vi "数据查询_数据查询.vi"() -> ()   [LabVIEW 2016]
uses:
  <vilib>/Utility/miscctls.llb/LVPointTypeDef.ctl
  <vilib>/Utility/miscctls.llb/LVRowAndColumnUnsignedTypeDef.ctl
  <userlib>/_OpenG.lib/array/array.llb/Sort 2D Array (String)__ogtk.vi
  <userlib>/_OpenG.lib/array/array.llb/Sort 1D Array (I32)__ogtk.vi
  <vilib>/addons/database/_DB Variant To Data/Database Variant To Data.xnode
panel:
  out "布尔文本.文本":string
  in  "数值":dbl=100.0 caption="显示条数"
  in  "单选按钮":T1(radio)
  in  "滚动条":i32(c297)
  in  "数组":string[](array[string])
  in  "导出":bool
  out "数据筛选_分钟小时":string(combo)="实时数据"
  out "数据筛选_工作类型":string(combo)="全部数据"
  out "连接的字符串":string
  out "选中数据表":string
  in  "查询":bool
  in  "结束日期":string="2050/01/01"
  in  "起始日期":string="2010/01/01"
  out "XY图":cluster{"data":timestamp[], "data":dbl[]}[](graph)
  in  "数据表":T2
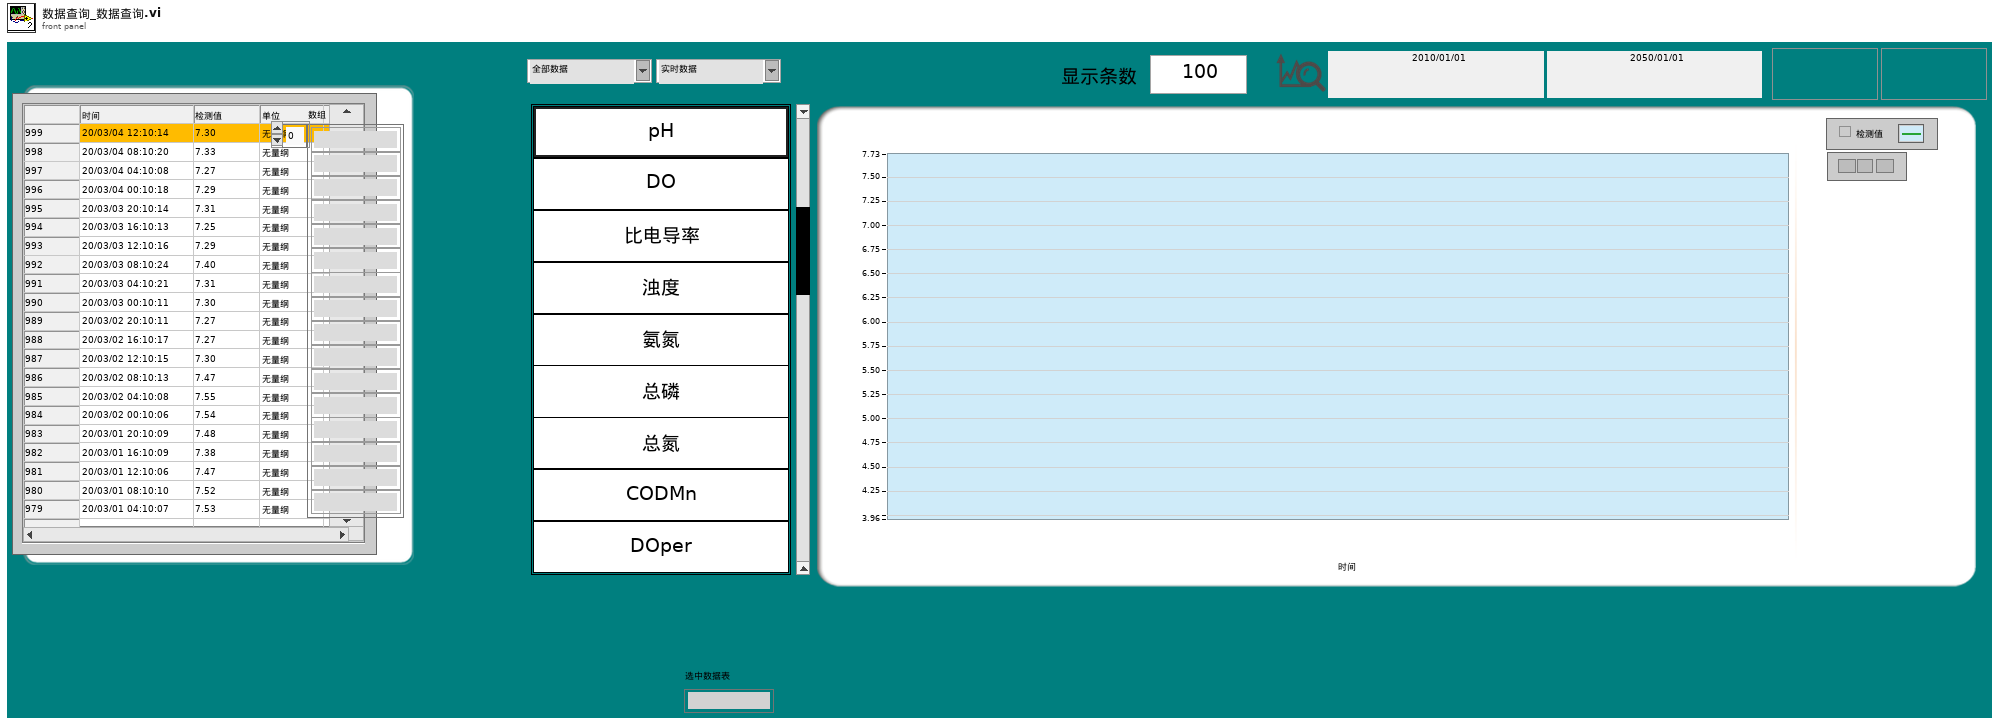
[diagram p1: front panel]
types:
  T1 = enum32{"单选选项1", "单选选项1 2", "单选选项1 3", "单选选项1 4", "单选选项1 5", "单选选项1 6", "单选选项1 7", "单选选项1 8", "单选选项1 9"}
  T2 = typedef "数据查询页列表框.ctl" = i32
  T3 = typedef "LVRowAndColumnUnsignedTypeDef.ctl" = cluster{"Row":u32, "Column":u32}
  T4 = typedef "LVPointTypeDef.ctl" = cluster{"Horizontal":i16, "Vertical":i16}
  T5 = enum8{"Enabled", "Disabled", "Disabled and Grayed Out"}
  T6 = typedef "LVPoint32TypeDef.ctl" = cluster{"Horizontal":i32, "Vertical":i32}
  T7 = typedef "LVPointDoubleTypeDef.ctl" = cluster{"Cursor X":dbl, "Cursor Y":dbl}
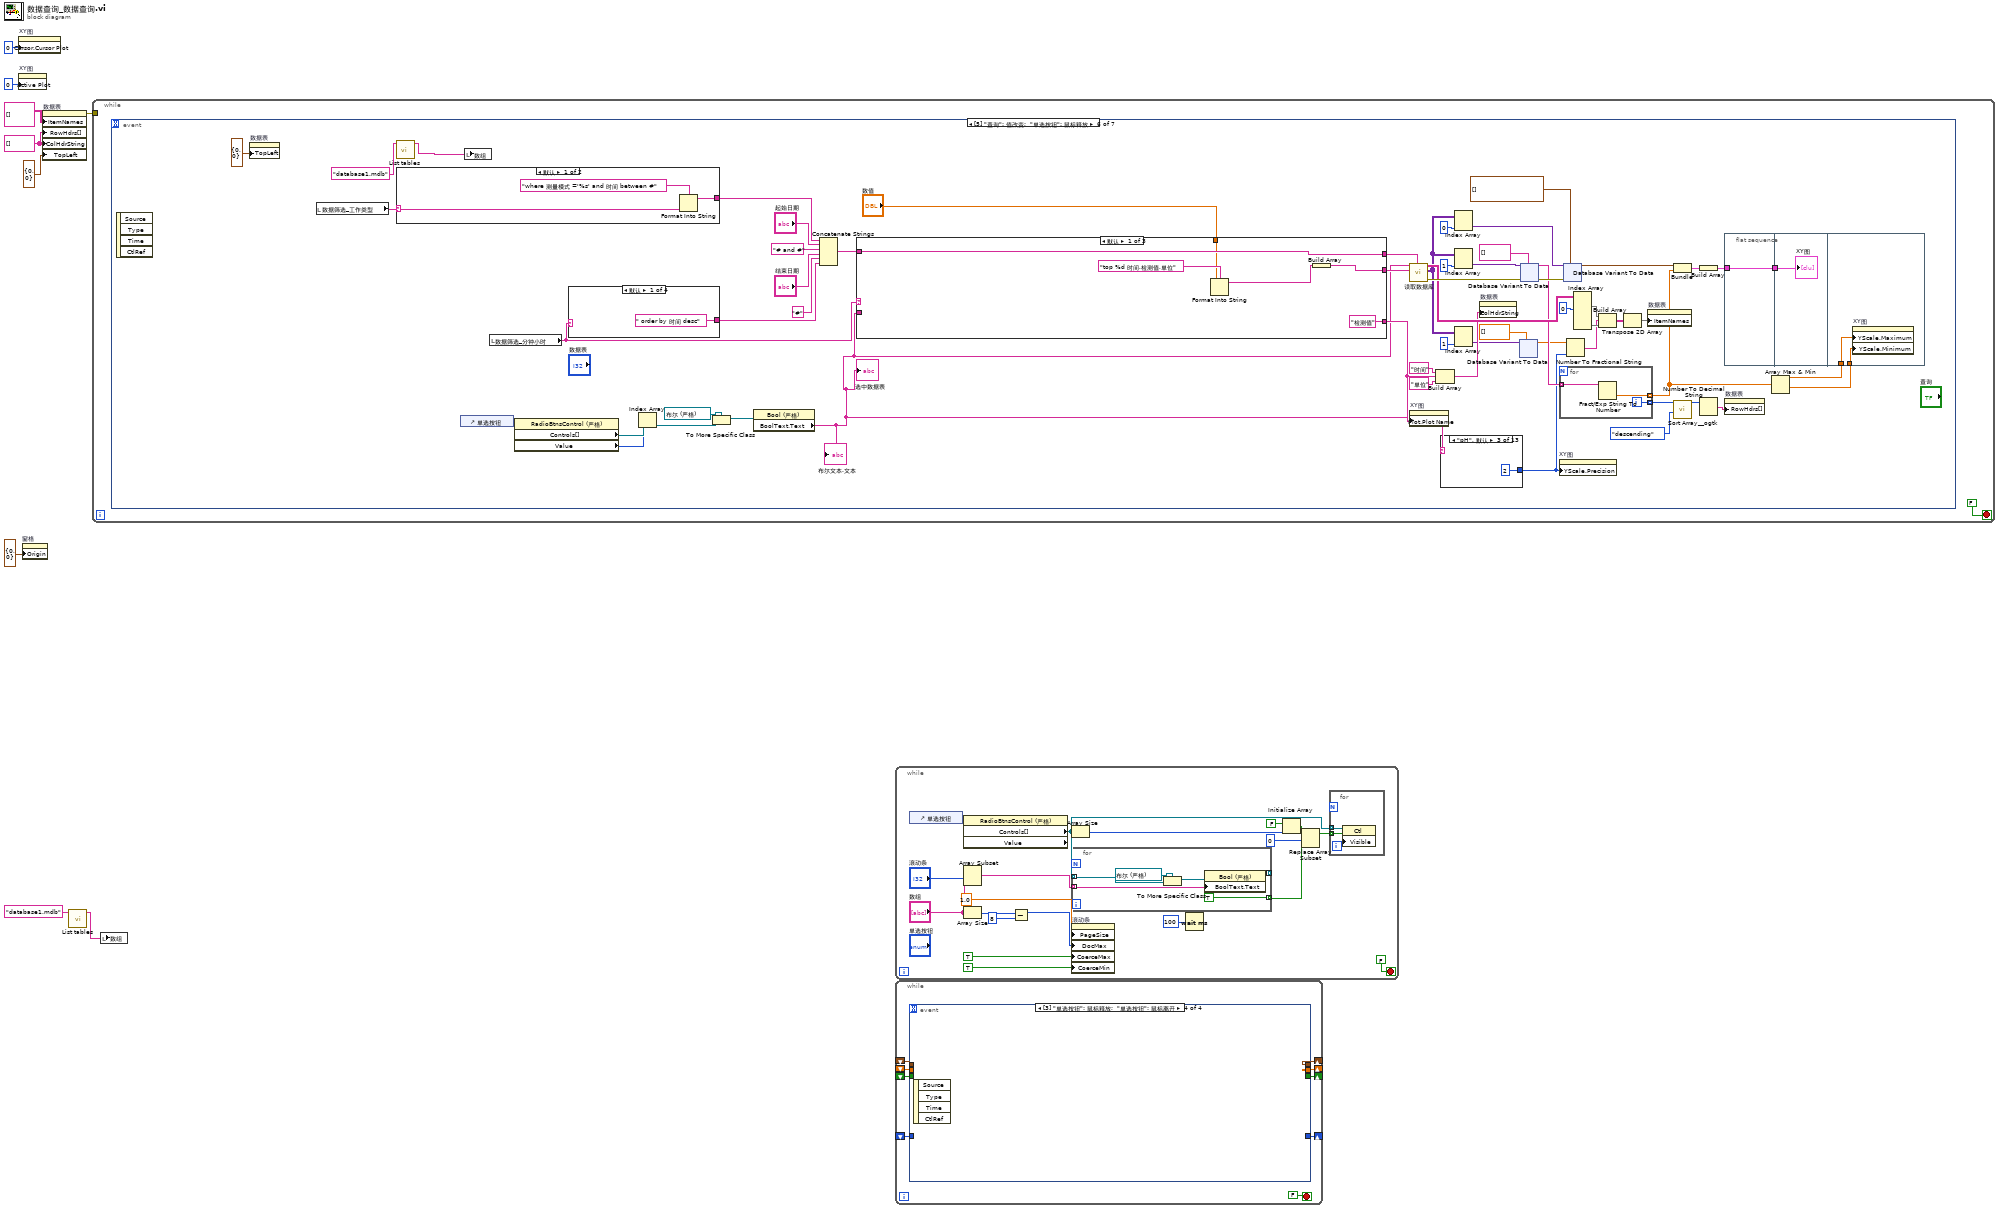
[diagram p0: block diagram]
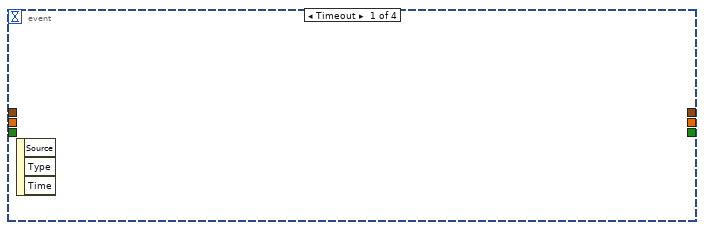
[diagram p2: hidden frame]
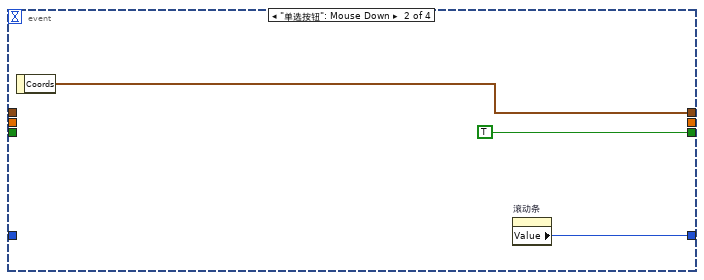
[diagram p3: hidden frame]
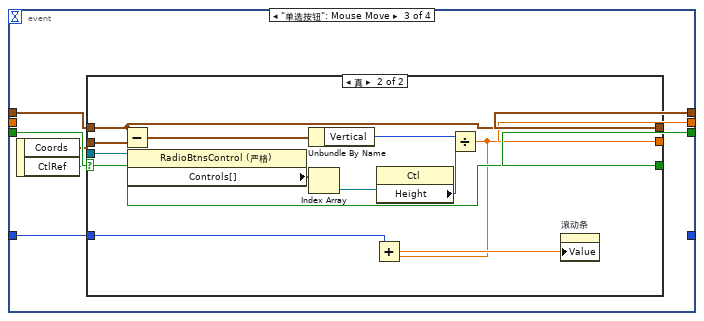
[diagram p4: hidden frame]
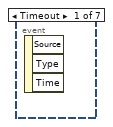
[diagram p6: hidden frame]
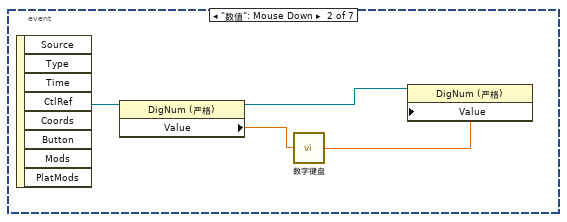
[diagram p7: hidden frame]
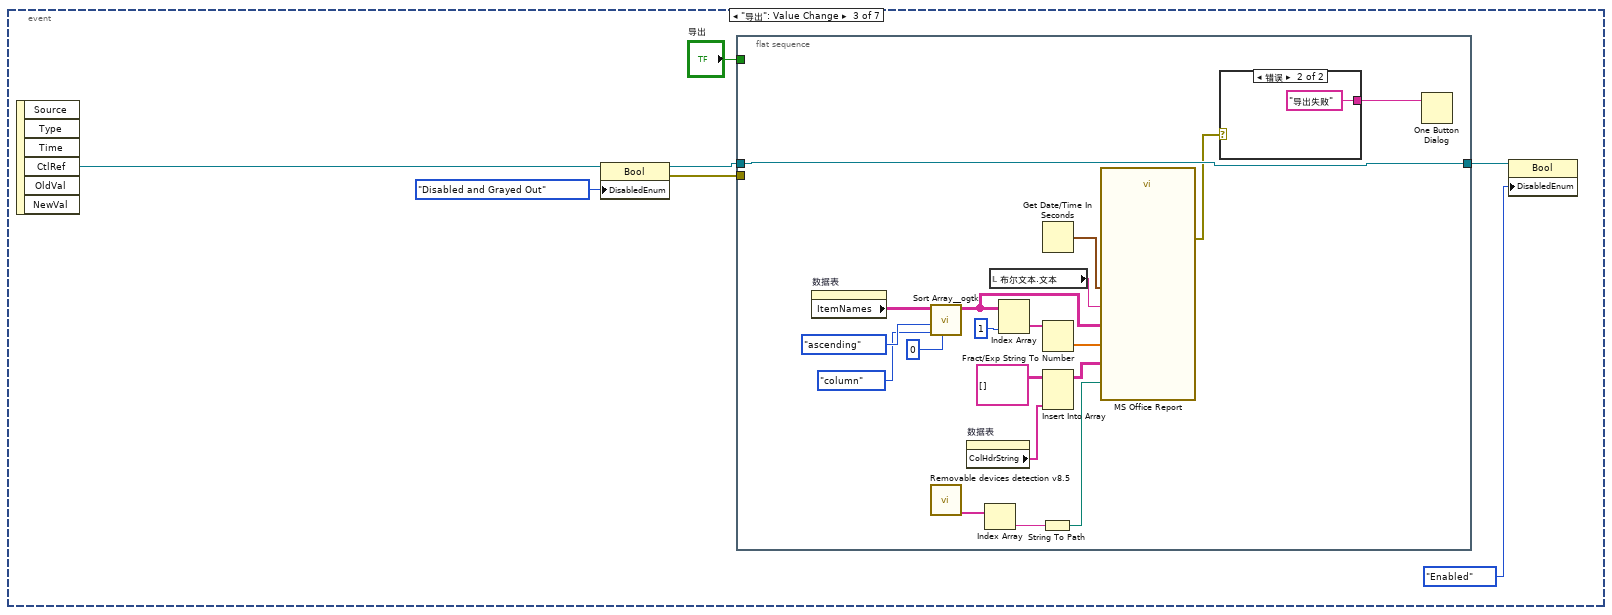
[diagram p8: hidden frame]
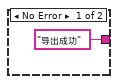
[diagram p9: hidden frame]
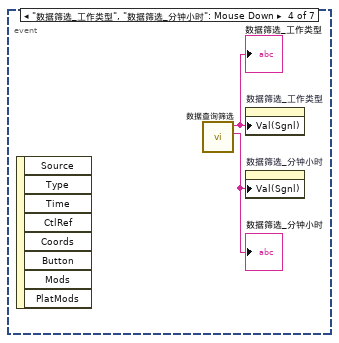
[diagram p10: hidden frame]
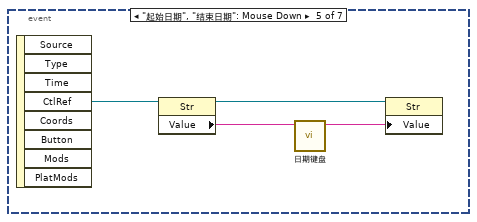
[diagram p11: hidden frame]
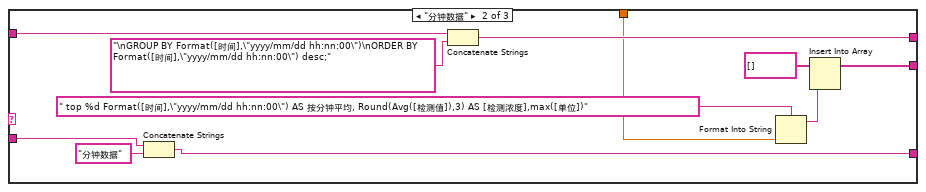
[diagram p12: hidden frame]
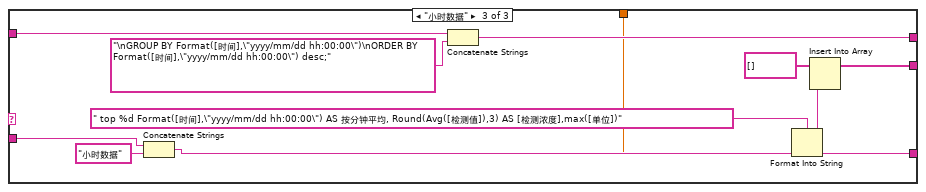
[diagram p13: hidden frame]
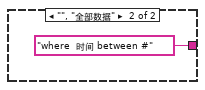
[diagram p17: hidden frame]
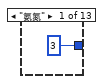
[diagram p18: hidden frame]
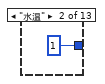
[diagram p19: hidden frame]
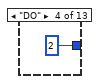
[diagram p20: hidden frame]
diagram:
  w3 = string[] [] ("行首字符串[]")
  n1 = property on="XY图" class="XYGraph (严格)"("Cursor.Cursor Plot"=0 ("游标.游标关联曲线")) -> ()  [unwired: 2 in, 2 out]
  n2 = property on="XY图" class="XYGraph (严格)"("Active Plot"=u32 0 ("活动曲线")) -> ()  [unwired: 2 in, 2 out]
  n3 = property on="窗格" class="Pane"("Origin"=T4 {"Horizontal"=0, "Vertical"=0} ("原点")) -> ()  [unwired: 2 in, 2 out]
  n4 = property on="数据表" class="MCListbox (严格)"("ItemNames"=string[][] [] ("项名"), "RowHdrs[]"=w3, "ColHdrString"=w3, "TopLeft"=T3 {"Row"=0, "Column"=0} ("左上可见单元格")) -> (error out=w5:errorcluster)  [unwired: 2 in, 1 out]
  n5 = call "List tables.vi"("database"="database1.mdb") -> ("tables"=w1:string[])  [unwired: 9 in, 1 out]
  n6 = while {
    tunnel: w5 -> [_]
    stop <- FALSE stop-if-true
    n7 = event shown="[5] \"查询\": 值改变;  \"单选按钮\": 鼠标释放" {
      selector: _ -> [_ _ _ _ _ _ _]
      dyn-events: _ -> [_ _ _ _ _ _ _]
      timeout: _ -> [_ _ _ _ _ _ _]
      event Timeout {
        n8 = event-data() -> ()  [unwired: 1 in, 3 out]
      }
      event "数值": Mouse Down {
        n9 = event-data() -> ("CtlRef"=w14:refnum<vi>)  [unwired: 1 in, 7 out]
        n10 = property class="DigNum (严格)"(reference=w14) -> (reference out=w13:refnum<vi>, "Value"=w12:dbl)  [unwired: 1 in, 1 out]
        n11 = call "数字键盘.vi"("OldNumber"=w12) -> ("NewNumber"=w11:sgl)
        n12 = property class="DigNum (严格)"(reference=w13, "Value"=w11) -> ()  [unwired: 1 in, 2 out]
      }
      event "导出": Value Change {
        n13 = event-data() -> ("CtlRef"=w21:refnum<vi>)  [unwired: 1 in, 5 out]
        n14 = property class="Bool"(reference=w21, "DisabledEnum"=T5."Disabled and Grayed Out" ("禁用")) -> (reference out=w18:refnum<vi>, error out=w19:errorcluster)  [unwired: 1 in]
        n15 = flat-sequence {
          tunnel: w19 -> [_]
          tunnel: [w31] -> w17
          tunnel: w18 -> [w31]
          tunnel: "导出" -> [_]
          frame #0 {
            n16 = property on="数据表" class="MCListbox (严格)"() -> ("ItemNames"=w22:string[][])  [unwired: 2 in, 2 out]
            n17 = call-poly <userlib>:"Sort Array__ogtk.vi"("Column/Row to Sort By"=u32 0, "Sort By in"=enum16{"row", "column"}."column", "Order"=enum16{"ascending", "descending"}."ascending", "Array in"=w22) -> ("Sorted Array out"=w38:string[][])  [unwired: 4 in, 3 out]
            n18 = call "Removable devices detection v8.5.vi"() -> ("Removable"=w28:string[])  [unwired: 4 out]
            n19 = property on="数据表" class="MCListbox (严格)"() -> ("ColHdrString"=w24:string[])  [unwired: 2 in, 2 out]
            n20 = Index Array(array=w28) -> (element=w27:string)  [unwired: 1 in]
            n21 = local read "布尔文本.文本"() -> (w32:string)
            n22 = Index Array(array=w38, index (col)=1 ("禁用的索引 (列)")) -> (element=w34:string[])  [unwired: 1 in]
            n23 = String To Path(string=w27) -> (path=w26:path)
            n24 = Get Date/Time In Seconds() -> (seconds since 1Jan1904=w40:timestamp)
            n25 = Fract/Exp String To Number(string=w34) -> (number=w33:dbl[])  [unwired: 3 in, 1 out]
            n26 = Insert Into Array(array=string[][] [], new element=w24) -> (w23:string[][])  [unwired: 2 in]
            n27 = call "MS Office Report"("Path to Save Report"=w26, "导出日期"=w40, "监测参数"=w32, "数据输入"=w38, "图表输入"=w33, "字段定义"=w23) -> ("error out"=w30:errorcluster)  [unwired: 20 in, 1 out]
            n28 = case shown="错误" w30 {
              tunnel: ["导出成功" ("消息") "导出失败" ("消息")] -> w29
              frame No Error {
              }
              frame Error {
              }
            }
            n29 = One Button Dialog(message=w29) -> ()  [unwired: 1 in, 1 out]
          }
        }
        n30 = property class="Bool"(reference=w17, "DisabledEnum"=T5."Enabled" ("禁用")) -> ()  [unwired: 1 in, 2 out]
      }
      event "数据筛选_工作类型", "数据筛选_分钟小时": Mouse Down {
        n31 = event-data() -> ()  [unwired: 1 in, 8 out]
        n32 = call "数据查询筛选.vi"() -> ("分钟小时"=w44:string, "工作类型"=w43:string)  [unwired: 10 in]
        "数据筛选_工作类型" <- w43
        "数据筛选_分钟小时" <- w44
        n33 = property on="数据筛选_工作类型" class="CmbBox"("Val(Sgnl)"=w43) -> ()  [unwired: 2 in, 2 out]
        n34 = property on="数据筛选_分钟小时" class="CmbBox"("Val(Sgnl)"=w44) -> ()  [unwired: 2 in, 2 out]
      }
      event "起始日期", "结束日期": Mouse Down {
        n35 = event-data() -> ("CtlRef"=w48:refnum<vi>)  [unwired: 1 in, 7 out]
        n36 = property class="Str"(reference=w48) -> (reference out=w46:refnum<vi>, "Value"=w47:string)  [unwired: 1 in, 1 out]
        n37 = call "日期键盘.vi"("原值"=w47) -> ("x+y"=w45:string)  [unwired: 10 in]
        n38 = property class="Str"(reference=w46, "Value"=w45) -> ()  [unwired: 1 in, 2 out]
      }
      event "查询": Value Change; "单选按钮": Mouse Up {
        n39 = event-data() -> ()  [unwired: 1 in, 4 out]
        n40 = property on="数据表" class="MCListbox (严格)"("TopLeft"=T3 {"Row"=0, "Column"=0} ("左上可见单元格")) -> ()  [unwired: 2 in, 2 out]
        n41 = local read "数据筛选_工作类型"() -> (w71:string)
        n42 = call "List tables.vi"("database"="database1.mdb") -> ("tables"=w50:string[])  [unwired: 9 in, 1 out]
        n43 = case shown="默认" w71 {
          selector: w71 -> [w139 _]
          tunnel: [w137 "where  时间 between #" ("condition")] -> w70
          frame Default {
            n44 = Format Into String(format string="where 测量模式 ='%s' and 时间 between #" ("condition"), w139) -> (resulting string=w137:string)  [unwired: 2 in, 1 out]
          }
          frame "", "全部数据" {
          }
        }
        n45 = control-ref of="单选按钮"() -> (w55:refnum<vi>)
        n46 = local write "数组"(w50) -> ()
        n47 = local read "数据筛选_分钟小时"() -> (w67:string)
        n48 = property class="RadioBtnsControl (严格)"(reference=w55) -> ("Controls[]"=w54:refnum<vi>[], "Value"=w53:T1)  [unwired: 1 in, 2 out]
        n49 = case shown="默认" w67 {
          tunnel: [" order by 时间 desc" ("字符串") _ _ _] -> w69
          frame Default {
          }
          frame "分钟数据" {
          }
          frame "小时数据" {
          }
          frame "真" {
          }
        }
        n50 = Index Array(array=w54, index=w53) -> (element=w52:refnum<vi>)
        n51 = To More Specific Class(target class=refnum<vi> refnum ("单选选项1"), reference=w52) -> (specific class reference=w57:refnum<vi>)  [unwired: 1 in, 1 out]
        n52 = property class="Bool (严格)"(reference=w57) -> ("BoolText.Text"=w51:string)  [unwired: 1 in, 2 out]
        "选中数据表" <- w51
        "布尔文本.文本" <- w51
        n53 = Concatenate Strings(w70, "起始日期", "# and #" ("condition"), "结束日期", "#" ("condition"), w69) -> (w68:string)
        n54 = case shown="默认" w67 {
          tunnel: [w112 w123 w131] -> w65
          tunnel: w68 -> [w113 w122 w133]
          tunnel: [w113 w121 w132] -> w66
          tunnel: ["检测值" w117 w128] -> w64
          tunnel: w51 -> [_ w118 w130]
          tunnel: "数值" -> [w108 w114 w125]
          frame Default {
            n55 = Format Into String(format string="top %d 时间,检测值,单位" ("格式字符串"), w108) -> (resulting string=w110:string)  [unwired: 2 in, 1 out]
            n56 = Build Array(w110) -> (w112:string[])
          }
          frame "分钟数据" {
            n57 = Concatenate Strings(w118, "分钟数据" ("字符串")) -> (w117:string)
            n58 = Concatenate Strings(w122, "\nGROUP BY Format([时间],\"yyyy/mm/dd hh:nn:00\")\nORDER BY Format([时间],\"yyyy/mm/dd hh:nn:00\") desc;" ("字符串")) -> (w121:string)
            n59 = Format Into String(format string=" top %d Format([时间],\"yyyy/mm/dd hh:nn:00\") AS 按分钟平均, Round(Avg([检测值]),3) AS [检测浓度],max([单位])" ("新元素/子数组"), w114) -> (resulting string=w115:string)  [unwired: 2 in, 1 out]
            n60 = Insert Into Array(array=string[] [] ("显示项"), new element=w115) -> (w123:string[])  [unwired: 1 in]
          }
          frame "小时数据" {
            n61 = Concatenate Strings(w130, "小时数据" ("字符串")) -> (w128:string)
            n62 = Concatenate Strings(w133, "\nGROUP BY Format([时间],\"yyyy/mm/dd hh:00:00\")\nORDER BY Format([时间],\"yyyy/mm/dd hh:00:00\") desc;" ("字符串")) -> (w132:string)
            n63 = Format Into String(format string=" top %d Format([时间],\"yyyy/mm/dd hh:00:00\") AS 按分钟平均, Round(Avg([检测值]),3) AS [检测浓度],max([单位])" ("新元素/子数组"), w125) -> (resulting string=w126:string)  [unwired: 2 in, 1 out]
            n64 = Insert Into Array(array=string[] [] ("显示项"), new element=w126) -> (w131:string[])  [unwired: 1 in]
          }
        }
        n65 = call "读取数据库.vi"("condition"=w66, "显示项"=w65, "组合框"=w51) -> ("error out"=w98:errorcluster, "data"=w83:variant[][], "表格"=w92:string[][])  [unwired: 5 in, 1 out]
        n66 = property on="XY图" class="XYGraph (严格)"("Plot.Plot Name"=w64) -> ()  [unwired: 2 in, 2 out]
        n67 = Build Array("时间", w64, "单位" ("元素")) -> (w87:string[])
        n68 = case shown="\"pH\", 默认" w51 {
          tunnel: [i16 3 ("精度(6)") i16 1 ("精度(6)") i16 2 ("精度(6)") i16 2 ("精度(6)") i16 2 ("精度(6)") i16 2 ("精度(6)") i16 2 ("精度(6)") i16 2 ("精度(6)") i16 2 ("精度(6)") i16 3 ("精度(6)") i16 2 ("精度(6)") i16 2 ("精度(6)") i16 2 ("精度(6)")] -> w72
          frame "氨氮" {
          }
          frame "水温" {
          }
          frame "pH", Default {
          }
          frame "DO" {
          }
          frame "DOper" {
          }
          frame "电导率" {
          }
          frame "浊度" {
          }
          frame "藻密度" {
          }
          frame "叶绿素a" {
          }
          frame "总磷" {
          }
          frame "总氮" {
          }
          frame "CodCr" {
          }
          frame "CodMn" {
          }
        }
        n69 = Index Array(array=w83, index (col)=0 ("禁用的索引 (列)")) -> (element=w101:variant[])  [unwired: 1 in]
        n70 = Index Array(array=w83, index (col)=1 ("禁用的索引 (列)")) -> (element=w99:variant[])  [unwired: 1 in]
        n71 = Index Array(array=w83, index (col)=1 ("禁用的索引 (列)")) -> (element=w81:variant[])  [unwired: 1 in]
        n72 = property on="数据表" class="MCListbox (严格)"("ColHdrString"=w87) -> ()  [unwired: 2 in, 2 out]
        n73 = xnode "Database Variant To Data"("database variant"=w81, "type"=sgl[] []) -> ("data"=w79:sgl[])  [unwired: 1 in, 1 out]
        n74 = xnode "Database Variant To Data"("database variant"=w99, "error in (no error)"=w98, "type"=string[] []) -> ("data"=w86:string[], "error out"=w97:errorcluster)
        n75 = for {
          tunnel: w86 -> [w194] mode=indexing
          tunnel: [w193] -> w75 mode=indexing
          tunnel: [w192] -> w61 mode=indexing
          i -> [w192]
          n76 = Fract/Exp String To Number(string=w194) -> (number=w193:dbl)  [unwired: 3 in, 1 out]
        }
        n77 = property on="XY图" class="XYGraph (严格)"("YScale.Precision"=w72) -> ()  [unwired: 2 in, 2 out]
        n78 = xnode "Database Variant To Data"("database variant"=w101, "error in (no error)"=w97, "type"=timestamp[] []) -> ("data"=w93:timestamp[])  [unwired: 1 out]
        n79 = Number To Fractional String(number=w79, precision (6)=w72) -> (F-format string=w78:string[])  [unwired: 2 in]
        n80 = Index Array(array=w92, index (col) #1=0 ("禁用的索引 (列)")) -> (element #1=w90:string[], element #3=w84:string[])  [unwired: 5 in, 1 out]
        n81 = Build Array(w90, w78, w84) -> (w89:string[][])
        n82 = Transpose 2D Array(2D array=w89) -> (transposed array=w62:string[][])
        n83 = property on="数据表" class="MCListbox (严格)"("ItemNames"=w62) -> ()  [unwired: 2 in, 2 out]
        n84 = Bundle("data"=w93, w75) -> (w94:cluster{"data":timestamp[], dbl[]})  [unwired: 1 in]
        n85 = call-poly <userlib>:"Sort Array__ogtk.vi"("Order"=enum16{"ascending", "descending"}."descending", "Array in"=w61) -> ("Sorted Array out"=w59:i32[])  [unwired: 8 in, 1 out]
        n86 = Build Array(w94) -> (w95:cluster{"data":timestamp[], dbl[]}[])
        n87 = Number To Decimal String(number=w59) -> (decimal integer string=w63:string[])  [unwired: 1 in]
        n88 = flat-sequence {
          tunnel: [w195] -> w96
          tunnel: w95 -> [w195]
          tunnel: w96 -> [w196]
          tunnel: w74 -> [w198]
          tunnel: w73 -> [w197]
          frame #0 {
          }
          frame #1 {
            "XY图" <- w196
          }
          frame #2 {
            n89 = property on="XY图" class="XYGraph (严格)"("YScale.Maximum"=w198, "YScale.Minimum"=w197) -> ()  [unwired: 2 in, 2 out]
          }
        }
        n90 = property on="数据表" class="MCListbox (严格)"("RowHdrs[]"=w63) -> ()  [unwired: 2 in, 2 out]
        n91 = Array Max & Min(array=w75) -> (max value=w74:dbl, min value=w73:dbl)  [unwired: 2 out]
      }
      event "XY图": Mouse Move {
        w293 = "   " ("字符串")
        n92 = event-data() -> ("CtlRef"=w303:refnum<vi>, "Coords"=w302:T6)  [unwired: 1 in, 3 out]
        n93 = invoke class="XYGraph (严格)" method="Map Coords To XY"(reference=w303, "Coords"=w302) -> (reference out=w301:refnum<vi>, error out=w298:errorcluster, "XY"=w300:cluster{"X":dbl, "Y":dbl})  [unwired: 5 in, 4 out]
        n94 = property class="XYGraph (严格)"(reference=w301, error in=w298, "Cursor.Cursor Position"=w300) -> (error out=w299:errorcluster)  [unwired: 1 out]
        n95 = property on="XY图" class="XYGraph (严格)"(error in=w299) -> ("Cursor.Cursor Position"=w296:T7, "YScale.Precision"=w289:u8)  [unwired: 1 in, 2 out]
        n96 = Unbundle(w296) -> ("Cursor X"=w295:dbl, "Cursor Y"=w292:dbl)
        n97 = property on="XY图" class="XYGraph (严格)"() -> ("Plot.Plot Name"=w290:string)  [unwired: 2 in, 2 out]
        n98 = Number To Fractional String(number=w292, precision (6)=w289) -> (F-format string=w291:string)  [unwired: 2 in]
        n99 = Format Date/Time String(seconds (now)=w295) -> (date/time string=w294:string)  [unwired: 2 in]
        n100 = Concatenate Strings(w290, w293, w294, w293, w291) -> (→"连接的字符串":string)
      }
    }
  }
  n101 = local write "数组"(w1) -> ()
  n102 = while {
    stop <- FALSE stop-if-true
    n103 = control-ref of="单选按钮"() -> (w322:refnum<vi>)
    n104 = property class="RadioBtnsControl (严格)" props=["Controls[]", "Value"](reference=w322) -> ("Controls[]"=w306:refnum<vi>[])  [unwired: 1 in, 3 out]
    n105 = Array Subset(array="数组", index="滚动条") -> (w318:string[])  [unwired: 1 in]
    n106 = Array Size(array="数组") -> (size(s)=w320:i32)
    n107 = Subtract(x=w320, y=8) -> (x-y=w305:i32)
    n108 = Array Size(array=w306) -> (size(s)=w314:i32)
    n109 = for {
      tunnel: w318 -> [w327] mode=indexing
      tunnel: w306 -> [w330] mode=indexing
      tunnel: [w326] -> _ mode=indexing
      tunnel: [TRUE ("可见")] -> w312 mode=indexing
      n110 = To More Specific Class(target class=refnum<vi> refnum ("单选选项1"), reference=w330) -> (specific class reference=w329:refnum<vi>)  [unwired: 1 in, 1 out]
      n111 = property class="Bool (严格)"(reference=w329, "BoolText.Text"=w327) -> (reference out=w326:refnum<vi>)  [unwired: 1 in, 1 out]
    }
    n112 = property on="滚动条" class="Scroll (严格)"("PageSize"=1.0 ("页大小"), "DocMax"=w305, "CoerceMax"=TRUE ("强制最大值"), "CoerceMin"=TRUE ("强制最小值")) -> ()  [unwired: 2 in, 2 out]
    n113 = Wait (ms)(milliseconds to wait=u32 100 ("等待时间（毫秒）")) -> ()  [unwired: 1 out]
    n114 = Initialize Array(FALSE, w314) -> (w313:bool[])
    n115 = Replace Array Subset(array=w313, new element=w312, index=0 ("索引")) -> (w310:bool[])
    n116 = for {
      tunnel: w306 -> [w324] mode=indexing
      tunnel: w310 -> [w323] mode=indexing
      n117 = property class="Ctl"(reference=w324, "Visible"=w323) -> ()  [unwired: 1 in, 2 out]
    }
  }
  n118 = while {
    shift-right: [w338] -> _
    shift-left: _ -> [w337]
    shift-right: [w336] -> _
    shift-left: _ -> [w335]
    shift-right: [w334] -> _
    shift-left: _ -> [w333]
    shift-right: [w332] -> _
    shift-left: _ -> [w331]
    stop <- FALSE stop-if-true
    n119 = event shown="[3] \"单选按钮\": 鼠标释放;  \"单选按钮\": 鼠标离开" {
      selector: _ -> [_ _ _ _]
      dyn-events: _ -> [_ _ _ _]
      timeout: _ -> [_ _ _ _]
      tunnel: [_ w342 w347 _] -> w338
      tunnel: w337 -> [_ _ w349 _]
      tunnel: [_ TRUE w345 _] -> w336
      tunnel: w335 -> [_ _ w350 _]
      tunnel: [_ _ w344 _] -> w334
      tunnel: w333 -> [_ _ _ _]
      tunnel: [_ w340 _ _] -> w332
      tunnel: w331 -> [_ _ w343 _]
      event Timeout {
        n120 = event-data() -> ()  [unwired: 1 in, 3 out]
      }
      event "单选按钮": Mouse Down {
        n121 = event-data() -> ("Coords"=w342:T6)  [unwired: 1 in]
        n122 = property on="滚动条" class="Scroll (严格)"() -> ("Value"=w340:i32)  [unwired: 2 in, 2 out]
      }
      event "单选按钮": Mouse Move {
        n123 = event-data() -> ("Coords"=w348:T6, "CtlRef"=w346:refnum<vi>)  [unwired: 1 in]
        n124 = case shown="真" w350 {
          selector: w350 -> [w351 w364]
          tunnel: w349 -> [w352 w356]
          tunnel: w348 -> [_ w357]
          tunnel: [w352 w356] -> w347
          tunnel: w346 -> [_ w363]
          tunnel: [w351 w364] -> w345
          tunnel: [_ w354] -> w344
          tunnel: w343 -> [_ w353]
          frame False {
          }
          frame True {
            n125 = Subtract(x=w356, y=w357) -> (x-y=w362:T6)
            n126 = property class="RadioBtnsControl (严格)"(reference=w363) -> ("Controls[]"=w360:refnum<vi>[])  [unwired: 1 in, 2 out]
            n127 = Unbundle By Name(w362) -> ("Vertical"=w361:i32)
            n128 = Index Array(array=w360) -> (element=w359:refnum<vi>)  [unwired: 1 in]
            n129 = property class="Ctl"(reference=w359) -> ("Height"=w358:u32)  [unwired: 1 in, 2 out]
            n130 = Divide(x=w361, y=w358) -> (x/y=w354:dbl)
            n131 = Add(x=w353, y=w354) -> (x+y=w355:dbl)
            n132 = property on="滚动条" class="Scroll (严格)"("Value"=w355) -> ()  [unwired: 2 in, 2 out]
          }
        }
      }
      event "单选按钮": Mouse Up; "单选按钮": Mouse Leave {
        n133 = event-data() -> ()  [unwired: 1 in, 4 out]
      }
    }
  }
